vi "Exercicio 4.vi"() -> ()   [LabVIEW 2020]
uses:
  <vilib>/MakerHub/LINX/Public/Peripherals/Analog/Analog Read 1 Chan.vi
  <vilib>/MakerHub/LINX/Public/Peripherals/PWM/PWM Set Duty Cycle 1 Chan.vi
  <vilib>/MakerHub/LINX/Public/Peripherals/Analog/Analog Read N Chans.vi
  <vilib>/MakerHub/LINX/Private/Local IO/LinxAnalogRead.vi
  <vilib>/MakerHub/LINX/Public/Utilities/Check Channel.vi
  <vilib>/MakerHub/LINX/Public/Utilities/Open Serial.vi
  <vilib>/MakerHub/LINX/Private/Utilties/Generate Error.vi
  <vilib>/MakerHub/LINX/Public/Peripherals/PWM/PWM Set Duty Cycle N Chans.vi
  <vilib>/MakerHub/LINX/LMH-LINX.lvlib
  <vilib>/Analysis/NI_AALPro.lvlib
panel:
  out "Error Out":errorcluster
  in  "Sample Rate (s)":u32
  in  "Stop Button":bool
  out "Humidity Chart":dbl(graph)
  in  "Serial Port":refnum<visa-resource-name>
  out "Humidity (%)":dbl(slide) scale=0.0..100.0
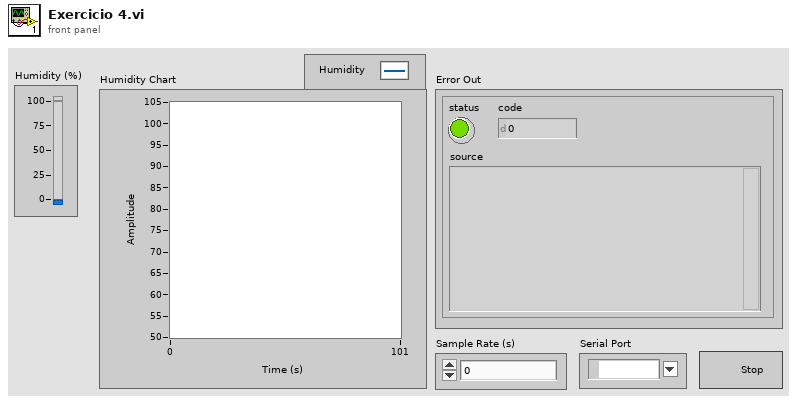
[diagram p1: front panel]
types:
  T1 = typedef "LMH-LINX.lvlib/LINX Ref.ctl" = cluster{"IO":T2, "Interface":T3, "LINX Device Config":T4}
  T2 = typedef "LMH-LINX.lvlib/Platform.ctl" = enum16{"Remote", "Local"}
  T3 = typedef "LMH-LINX.lvlib/Interface.ctl" = enum16{"Serial", "TCP"}
  T4 = typedef "LMH-LINX.lvlib/Device.lvlib/LINX Device Config.ctl" = cluster{"Interface":T3, "COM Port":refnum<visa-resource-name>, "TCP Configuration":T5, "Device Family":u8, "Device ID":u8, "Device Name":string, "TCP Ref":refnum<k5>, "Channels":T6}
  T5 = typedef "LMH-LINX.lvlib/Device.lvlib/TCP Config.ctl" = cluster{"IP Address":string, "Port":u16}
  T6 = typedef "LMH-LINX.lvlib/Channels.ctl" = cluster{"DI":u8[], "DO":u8[], "AI":u8[], "AO":u8[], "PWM":u8[], "QE":u8[], "UART":u8[], "I2C 2":u8[], "SPI":u8[], "CAN":u8[], "Servo":u8[], "AI Ref (V)":dbl, "AI Resolution (Bits)":u8, "AO Ref (V)":dbl, "AO Resolution (Bits)":u8}
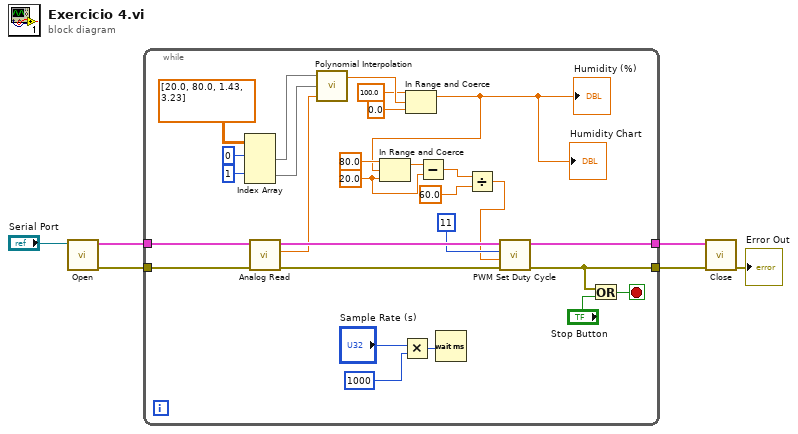
[diagram p0: block diagram]
diagram:
  n1 = call-poly <vilib>:"Open.vi"("Serial Port"="Serial Port") -> ("Error Out"=w2:errorcluster, "LINX Resource"=w5:T1)  [unwired: 8 in, 1 out]
  n2 = while {
    tunnel: w5 -> [w32]
    tunnel: [w30] -> w4
    tunnel: [w27] -> w3
    tunnel: w2 -> [w28]
    stop <- w33 stop-if-true
    w17 = 20.0 ("lower limit")
    n3 = Index Array(array=dbl[][] [[20.0, 80.0], [1.43, 3.23]], index (row) #1=0 ("index (row)"), index (row) #2=1 ("index (row)")) -> (element #1=w24:dbl[], element #2=w23:dbl[])  [unwired: 2 in]
    n4 = call-poly <vilib>:"Analog Read.vi"("Error In"=w28, "LINX Resource"=w32) -> ("Error Out"=w29:errorcluster, "Voltage"=w20:dbl, "LINX Resource"=w31:T1)  [unwired: 6 in, 1 out]
    n5 = call <vilib>:"Polynomial Interpolation.vi"("x value"=w20, "X"=w23, "Y"=w24) -> ("interpolation value"=w13:dbl)  [unwired: 2 out]
    n6 = Multiply(x="Sample Rate (s)", y=u32 1000) -> (x*y=w9:u32)
    n7 = In Range and Coerce(upper limit=100.0, x=w13, lower limit=0.0) -> (coerced(x)=w10:dbl)  [unwired: 1 out]
    "Humidity (%)" <- w10
    "Humidity Chart" <- w10
    n8 = In Range and Coerce(upper limit=80.0, x=w10, lower limit=w17) -> (coerced(x)=w18:dbl)  [unwired: 1 out]
    n9 = Subtract(x=w18, y=w17) -> (x-y=w15:dbl)
    n10 = Wait (ms)(milliseconds to wait=w9) -> ()  [unwired: 1 out]
    n11 = Divide(x=w15, y=60.0) -> (x/y=w14:dbl)
    n12 = call-poly <vilib>:"PWM Set Duty Cycle.vi"("Error In"=w29, "Duty Cycle (0-1)"=w14, "PWM Channel"=u8 11, "LINX Resource"=w31) -> ("Error Out"=w27:errorcluster, "LINX Resource"=w30:T1)  [unwired: 6 in]
    n13 = Or(x=w27, y="Stop Button") -> (x .or. y?=w33:bool)
  }
  n14 = call <vilib>:"Close.vi"("Error In"=w3, "LINX Resource"=w4) -> ("Error Out"=→"Error Out":errorcluster)  [unwired: 9 in]
